vi "Lmax.vi"(11 "Numeric":dbl) -> (3 "Lmax":dbl)   [LabVIEW 2020]
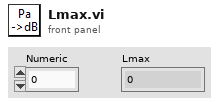
[diagram p1: front panel]
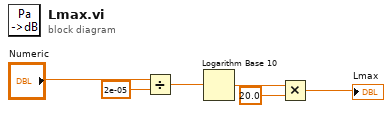
[diagram p0: block diagram]
diagram:
  n1 = Divide(x="Numeric", y=2e-05) -> (x/y=w4:dbl)
  n2 = Logarithm Base 10(1:w4) -> (0:w3:dbl)
  n3 = Multiply(x=w3, y=20.0) -> (x*y=→"Lmax":dbl)
